vi "zad2.vi"() -> ()   [LabVIEW 2018]
uses:
  <vilib>/sound2/lvsound2.llb/Sound Data Format.ctl
  <vilib>/sound2/lvsound2.llb/Sampling Mode.ctl
  <vilib>/sound2/lvsound2.llb/Sound Output Set Volume (Single).vi
  <vilib>/sound2/lvsound2.llb/Sound Output Write (DBL Single).vi
  <vilib>/measure/NI_MABase.lvlib
panel:
  out "Waveform Graph":waveform(dbl)(graph)
  in  "frequency":dbl(knob)=10.0 scale=20.0..2000.0
  in  "stop":bool
  in  "volume":dbl(slide)=100.0 scale=0.0..10.0
  in  "device ID":u32
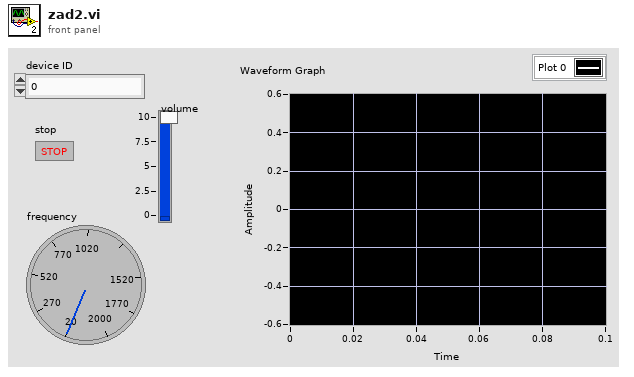
[diagram p1: front panel]
types:
  T1 = typedef "Sampling Mode.ctl" = i32
  T2 = typedef "Sound Data Format.ctl" = cluster{"sample rate (S/s)":dbl, "number of channels":i32, "bits per sample":i32}
  T3 = typedef "Sound Output Task ID.ctl" = u32
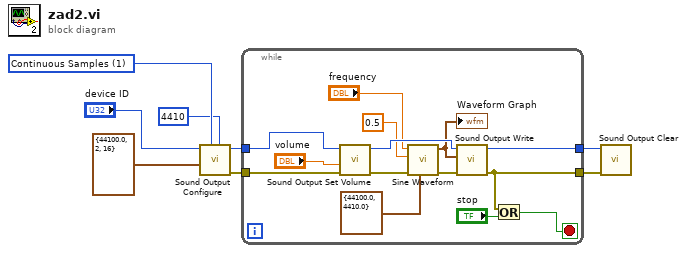
[diagram p0: block diagram]
diagram:
  w6 = T1 1 items=["Finite Samples", "Continuous Samples"] ("sample mode")
  n1 = call <vilib>:"Sound Output Configure.vi"("number of samples/ch"=4410, "sample mode"=w6, "sound format"=T2 {"sample rate (S/s)"=44100.0, "number of channels"=2, "bits per sample"=16}, "device ID"="device ID") -> ("error out"=w3:errorcluster, "task ID"=w4:T3)  [unwired: 6 in]
  n2 = while {
    tunnel: w4 -> [w22]
    tunnel: w3 -> [w21]
    tunnel: [w17] -> w2
    tunnel: [w16] -> w1
    stop <- w9 stop-if-true
    n3 = call-poly <vilib>:"Sound Output Set Volume.vi"("error in (no error)"=w21, "volume"="volume", "task ID"=w22) -> ("error out"=w10:errorcluster, "task ID out"=w19:T3)  [unwired: 7 in]
    n4 = call <vilib>:"Sine Waveform.vi"("sampling info"=cluster{"Fs":dbl, "#s":dbl} {"Fs"=44100.0, "#s"=4410.0}, "error in (no error)"=w10, "amplitude"=0.5, "frequency"="frequency") -> ("error out"=w12:errorcluster, "signal out"=w11:waveform(dbl))  [unwired: 6 in]
    "Waveform Graph" <- w11
    n5 = call-poly <vilib>:"Sound Output Write.vi"("error in (no error)"=w12, "data"=w11, "task ID"=w19) -> ("error out"=w17:errorcluster, "task ID out"=w16:T3)  [unwired: 7 in]
    n6 = Or(x=w17, y="stop") -> (x .or. y?=w9:bool)
  }
  n7 = call <vilib>:"Sound Output Clear.vi"("error in (no error)"=w2, "task ID"=w1) -> ()  [unwired: 9 in, 1 out]
